vi "Standard Setup.vi"(8 "error in (no error)":errorcluster, 11 "CCDCamera in":refnum<class "CCDCamera.lvclass">) -> (0 "error out":errorcluster, 3 "CCDCamera out":refnum<class "CCDCamera.lvclass">)   [LabVIEW 2018, in "CCDCamera.lvclass"]
uses:
  CCDCamera.lvclass
  <userlib>/atmcd32d.llb/HSSpeed_type typedef.ctl
  <userlib>/atmcd32d.llb/Shutter_mode typedef.ctl
  CCDCamera.lvclass/CCDCamera.ctl
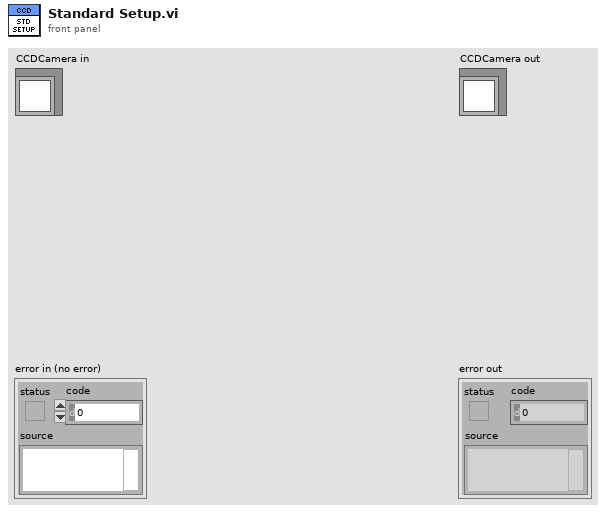
[diagram p1: front panel]
types:
  T1 = typedef "Shutter_mode typedef.ctl" = enum16{"Auto", "Open", "Close", "N/A (3)", "Open FVB Series", "Open Any Series"}
  T2 = typedef "HSSpeed_type typedef.ctl" = enum16{"EM Amp", "Conventional Amp"}
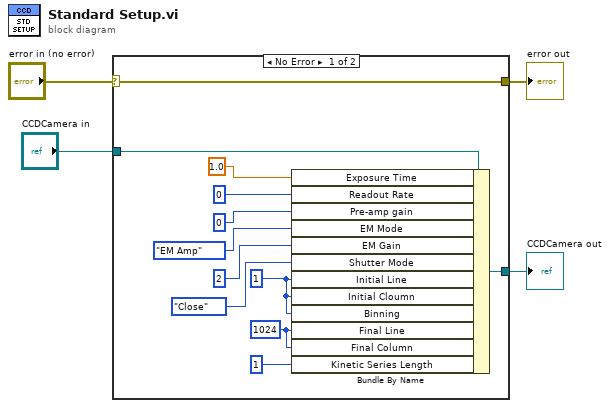
[diagram p0: block diagram]
diagram:
  n1 = case shown="No Error" "error in (no error)" {
    selector: "error in (no error)" -> [w16 w18]
    tunnel: [w16 w18] -> w2
    tunnel: [w14 w17] -> w1
    tunnel: "CCDCamera in" -> [w15 w17]
    frame No Error {
      w6 = u16 1024 ("Initial Line")
      w7 = u16 1 ("Initial Line")
      n2 = Bundle By Name(cluster=w15, "Exposure Time"=1.0, "Readout Rate"=u8 0, "Pre-amp gain"=u8 0, "EM Mode"=HSSpeed_type_typedef."EM Amp" ("type"), "EM Gain"=u16 2, "Shutter Mode"=Shutter_mode_typedef."Close" ("mode"), "Initial Line"=w7, "Initial Cloumn"=w7, "Binning"=w7, "Final Line"=w6, "Final Column"=w6, "Kinetic Series Length"=1) -> (w14:refnum<class "CCDCamera.lvclass">)
    }
    frame Error {
    }
  }
  "error out" <- w2
  "CCDCamera out" <- w1
